vi "Test Set Active Path.vi"(8 "error in (no error)":errorcluster) -> (0 "error out":errorcluster)   [LabVIEW 2019]
uses:
  Setting Database/Setting Database.lvclass
  C:/Program Files (x86)/National Instruments/LabVIEW 2019/vi.lib/JKI/JKI SMO/SMO/SMO.lvclass
  ObjectSettings/ObjectSettings.lvclass/ObjectSettings.ctl
  ObjectSettings/Accessors/Read Enabled.vi
  ObjectSettings/Accessors/Write Enabled.vi
  Path Settings/Path Settings.lvclass
  C:/Users/Albro/Documents/GitHub/AFM-Lithography/lvsrc/Classes/Settings/ObjectSettings/ObjectSettings.lvclass
  <vilib>/addons/_JKI Toolkits/Caraya/classes/Assert/Assert Equal Value_Variant.vi
  <vilib>/addons/_JKI Toolkits/Caraya/classes/Test/Test.lvclass
  <vilib>/addons/_JKI Toolkits/Caraya/classes/Assert/Assert.lvclass
  <vilib>/JKI/JKI SMO/SMO/SMO.lvclass
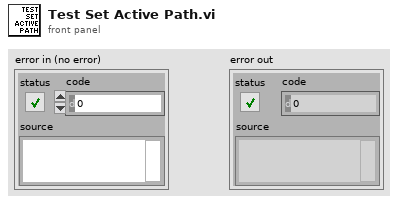
[diagram p1: front panel]
types:
  T1 = typedef "Setting Database.lvclass/PublicEvents--Cluster.ctl" = cluster{"NewActivePath":refnum<user-event>, "PathsUpdated":refnum<user-event>, "RectanglesUpdated":refnum<user-event>, "NewActiveRectangle":refnum<user-event>, "NewActiveFunnel":refnum<user-event>, "FunnelsUpdated":refnum<user-event>, "NewActiveDot":refnum<user-event>, "DotsUpdated":refnum<user-event>}
  T2 = typedef "Setting Database.lvclass/PrivateEvents--Setting Database.Refresh.ctl" = cluster{"Paths":string[], "Rectangles":string[], "Funnels":string[], "Dots":string[]}
  T3 = typedef "Setting Database.lvclass/PublicEvents--Setting Database.NewActivePath.ctl" = refnum<class "Path Settings.lvclass">
  T4 = typedef "Setting Database.lvclass/PublicEvents--Setting Database.PathsUpdated.ctl" = refnum<class "Path Settings.lvclass">[]
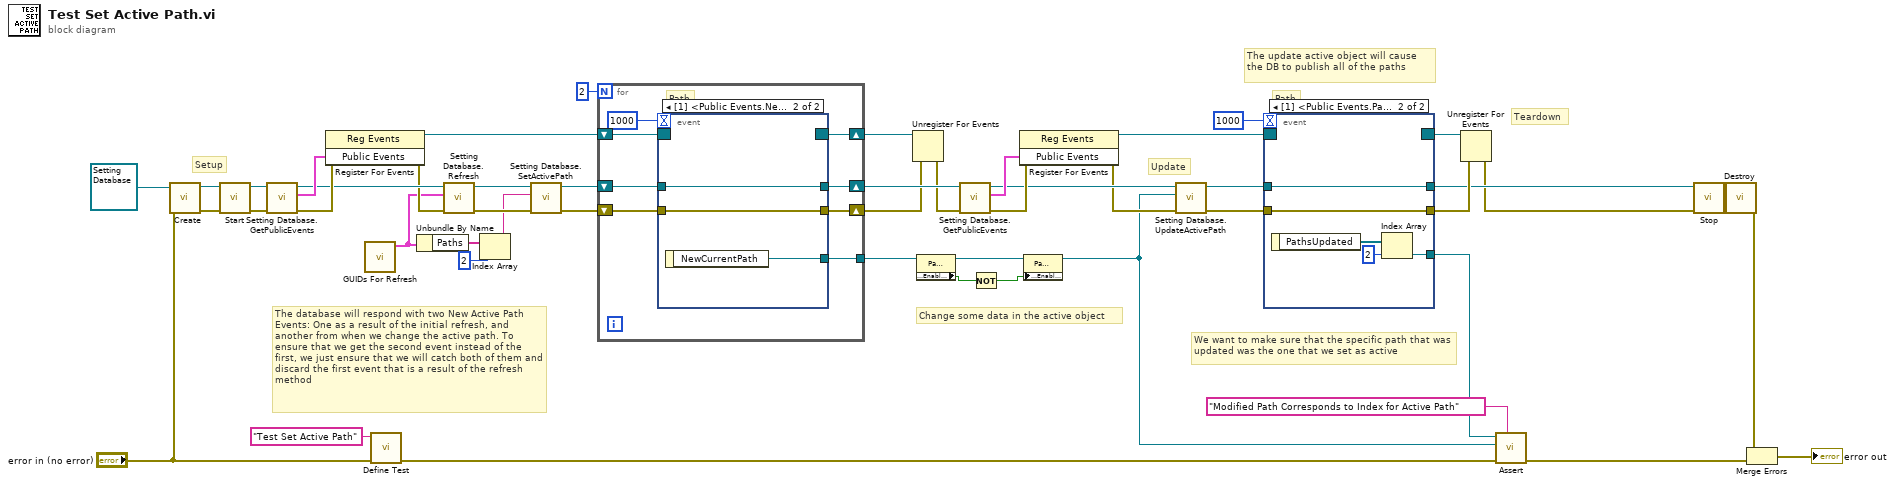
[diagram p0: block diagram]
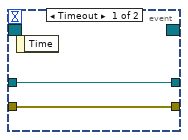
[diagram p2: hidden frame]
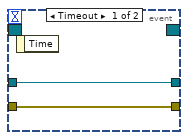
[diagram p3: hidden frame]
diagram:
  # "We want to make sure that the specific path that was updated was the one that we set as active"
  # "The update active object will cause the DB to publish all of the paths"
  # "Update"
  # "Change some data in the active object"
  # "The database will respond with two New Active Path Events: One as a result of the initial refresh, and another from when we change the active path. To ensure that we get the second event instead of the first, we just ensure that we will catch both of them and discard the first event that is a result of the refresh method"
  # "Path"
  # "Teardown"
  # "Setup"
  n1 = call <vilib>:"Create.vi"("error in (no error)"="error in (no error)", "SMO"=refnum<class "Setting Database.lvclass"> refnum ("Setting Database.lvclass")) -> ("error out"=w48:errorcluster, "SMO out"=w41:refnum<class "Setting Database.lvclass">)  [unwired: 7 in, 1 out]
  n2 = call <vilib>:"Start.vi"("error in (no error)"=w48, "SMO"=w41) -> ("error out"=w47:errorcluster, "SMO out"=w40:refnum<class "Setting Database.lvclass">)  [unwired: 8 in]
  n3 = call "Setting Database.GetPublicEvents.vi"("error in (no error)"=w47, "Setting Database"=w40) -> ("error out"=w45:errorcluster, "Public Events"=w37:T1, "Setting Database out"=w34:refnum<class "Setting Database.lvclass">)  [unwired: 7 in]
  n4 = register-events(error in=w45, w37) -> (reference out=w35:refnum<event-registration>, error out=w33:errorcluster)  [unwired: 1 in]
  n5 = call "GUIDs For Refresh.vi"() -> ("Initialize"=w6:T2)  [unwired: 10 in, 1 out]
  n6 = call <vilib>:"Define Test.vi"("error in (no error)"="error in (no error)", "Label (VI Title)"="Test Set Active Path") -> ("error out"=w50:errorcluster)  [unwired: 8 in, 1 out]
  n7 = Unbundle By Name(w6) -> ("Paths"=w5:string[])
  n8 = call "Setting Database.Refresh.vi"("error in (no error)"=w33, "Initialize"=w6, "Setting Database"=w34) -> ("error out"=w8:errorcluster, "Setting Database out"=w10:refnum<class "Setting Database.lvclass">)  [unwired: 7 in]
  n9 = Index Array(array=w5, index=2) -> (element=w3:string)
  n10 = call "Setting Database.SetActivePath.vi"("error in (no error)"=w8, "SetActivePath"=w3, "Setting Database"=w10) -> ("error out"=w7:errorcluster, "Setting Database out"=w9:refnum<class "Setting Database.lvclass">)  [unwired: 7 in]
  n11 = for {
    N: 2 -> [_]
    tunnel: [w51] -> w17
    shift-right: [w58] -> w38
    shift-left: w35 -> [w56]
    shift-right: [w53] -> w32
    shift-left: w9 -> [w55]
    shift-right: [w52] -> w31
    shift-left: w7 -> [w54]
    # "Path"
    n12 = event shown="[1] <Public Events.NewActivePath>: User Event" {
      selector: w56 -> [_ _]
      dyn-events: [_ _] -> w58
      timeout: 1000 -> [_ _]
      tunnel: [w60 w63] -> w52
      tunnel: w54 -> [w60 w63]
      tunnel: w55 -> [w59 w62]
      tunnel: [w59 w62] -> w53
      tunnel: [_ w61] -> w51
      event Timeout {
        n13 = event-data() -> ()  [unwired: 1 in, 1 out]
      }
      event User Event {
        n14 = event-data() -> ("NewCurrentPath"=w61:T3)  [unwired: 1 in]
      }
    }
  }
  n15 = Unregister For Events(event registration refnum=w38, error in=w31) -> (error out=w30:errorcluster)
  n16 = property on="Property Node" class="Path Settings.lvclass"(reference=w17) -> (reference out=w16:T3, "Accessors:Enabled"=w15:bool)  [unwired: 1 in, 1 out]
  n17 = call "Setting Database.GetPublicEvents.vi"("error in (no error)"=w30, "Setting Database"=w32) -> ("error out"=w28:errorcluster, "Public Events"=w29:T1, "Setting Database out"=w21:refnum<class "Setting Database.lvclass">)  [unwired: 7 in]
  n18 = Not(x=w15) -> (.not. x?=w14:bool)
  n19 = register-events(error in=w28, w29) -> (reference out=w24:refnum<event-registration>, error out=w19:errorcluster)  [unwired: 1 in]
  n20 = property on="Property Node" class="Path Settings.lvclass"(reference=w16, "Accessors:Enabled"=w14) -> (reference out=w13:T3)  [unwired: 1 in, 1 out]
  n21 = call "Setting Database.UpdateActivePath.vi"("error in (no error)"=w19, "UpdateCurrentPath"=w13, "Setting Database"=w21) -> ("error out"=w18:errorcluster, "Setting Database"=w20:refnum<class "Setting Database.lvclass">)  [unwired: 7 in]
  n22 = event shown="[1] <Public Events.PathsUpdated>: User Event" {
    selector: w24 -> [_ _]
    dyn-events: [_ _] -> w25
    timeout: 1000 -> [_ _]
    tunnel: [w65 w70] -> w27
    tunnel: w18 -> [w65 w70]
    tunnel: w20 -> [w64 w69]
    tunnel: [w64 w69] -> w23
    tunnel: [_ w67] -> w2
    event Timeout {
      n23 = event-data() -> ()  [unwired: 1 in, 1 out]
    }
    event User Event {
      n24 = event-data() -> ("PathsUpdated"=w68:T4)  [unwired: 1 in]
      n25 = Index Array(array=w68, index=2) -> (element=w67:refnum<class "Path Settings.lvclass">)
    }
  }
  n26 = Unregister For Events(event registration refnum=w25, error in=w27) -> (error out=w22:errorcluster)
  n27 = call-poly <vilib>:"Assert.vi"("Label"="Modified Path Corresponds to Index for Active Path", "error in (no error)"=w50, "Actual"=w13, "Expected"=w2) -> ("error out"=w1:errorcluster)  [unwired: 6 in, 1 out]
  n28 = call <vilib>:"Stop.vi"("error in (no error)"=w22, "SMO"=w23) -> ("error out"=w46:errorcluster, "SMO out"=w39:refnum<class "Setting Database.lvclass">)  [unwired: 8 in]
  n29 = call <vilib>:"Destroy.vi"("error in (no error)"=w46, "SMO"=w39) -> ("error out"=w44:errorcluster)  [unwired: 9 in]
  n30 = Merge Errors(w44, w1) -> (→"error out":errorcluster)
